vi "TIFF_6_Full_Write_Metadata.vi"(0 "Source File Image Path":path=path "C:/Users/Sebastien/Documents/GitHub/LABVIEW-Useful-codes/TIFF/Test_Image_1.tif", 5 "Destination Image Path":path=path "C:/Users/Sebastien/Documents/GitHub/LABVIEW-Useful-codes/TIFF/Test_Image_1_New.tif", 7 "User":T1(ring), 9 "XY resolution (nm)":string="125", 11 "error in (no error)":errorcluster) -> (15 "Error Out":errorcluster)   [LabVIEW 2025]
doc: "This software was created to prototype writing metadata to a TIFF file with a single image.\n\n<B>Usage:</B> This software is free to use, copy or plagiariaze. It is provided \"as-is\", and no technical support will be provided. The copyright is retained by NASA Marshall Space Flight Center.\n\n<B>Testing:</B> This software was tested by A) verifying that operations were completed successfully using LabVIEW 2009 on Windows XP, .NET version 4.0 and B) Windows Vista Microsoft Office Picture Manager was able to read and display the output file and C) Windows Vista Windows Photo Gallery was able to read and display the output file and the Description and D) Adobe Photoshop for Macintosh was able to correctly load and display the image and all the metadata.\n\n<B>Note:</B> This software requires .NET version 4.0\n\n<B>Warning:</B> This software will overwrite the destination file if it exists.\n\nThis software originally developed by:\nDerek Mayer\nBAE Systems - Technology Solutions & Services\n308 Voyager Way\nHuntsville, AL 35806\n(256) 890-8000\nwww.mevatec.com\nwww.baesystems.com/TSS\nSeptember 2010"
uses:
  TypeDef_FGV.ctl
  <vilib>/addons/_JKI.lib/Serialization/JSON/JKI JSON Serialization.lvlib
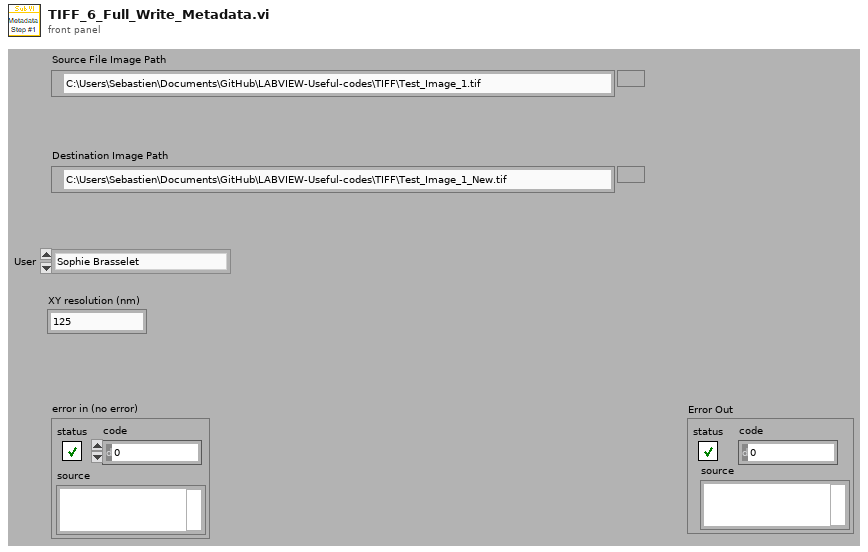
[diagram p1: front panel]
types:
  T1 = enum16{"Sophie Brasselet", "Jean-Jacques Honorine", "Sébastien Mailfert", "Manos Mavrakis"}
  T2 = typedef "TypeDef_FGV.ctl" = enum16{"Initialize", "Write", "Read", "Read_File", "Write_to_File"}
  T3 = typedef "TypeDef_Array_ChannelCluster.ctl" = cluster{"Laser":enum16{"640 nm", "561 nm"}, "Power":u8, "Exposure time":dbl, "Channel ON-OFF":bool, "Polar ON-OFF":bool, "FW 1":u16, "FW 2":u16}[]
  T4 = cluster{"Date/Time":string, "System model":string, "Software version":string, "Copyright":string, "User":string, "Description":string, "X resolution":string, "Y resolution":string, "Resolution unit":string}
  T5 = cluster{"Error":errorcluster, "Source Filestream":refnum<k24>, "TIFF Decoder":refnum<k24>, "TIFF Frames":refnum<k24>, "get_Item":refnum<k24>, "Bitmap Metadata":refnum<k24>, "New Encoder":refnum<k24>}
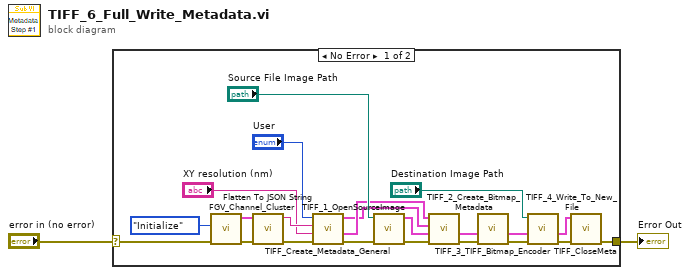
[diagram p0: block diagram]
diagram:
  n1 = case shown="No Error" "error in (no error)" {
    selector: "error in (no error)" -> [w12 w25]
    tunnel: [w14 w25] -> w1
    frame No Error {
      n2 = call "FGV_Channel_Cluster.vi"("error in"=w12, "Action"=TypeDef_FGV."Initialize") -> ("error out"=w11:errorcluster, "Channel_Cluster_Array OUT"=w10:T3)  [unwired: 8 in]
      n3 = call <vilib>:"Flatten To JSON String.vi"("error in"=w11, "Variant"=w10) -> ("error out"=w6:errorcluster, "JSON String"=w9:string)  [unwired: 8 in]
      n4 = call "TIFF_Create_Metadata_General.vi"("error in (no error)"=w6, "XY resolution (nm)"="XY resolution (nm)", "Description"=w9, "User"="User") -> ("error out"=w5:errorcluster, "Metadata OUT"=w4:T4, "Taggs"=w3:T4)  [unwired: 5 in]
      n5 = call "TIFF_1_OpenSourceImage.vi"("error in (no error)"=w5, "Source File Image Path"="Source File Image Path") -> ("Error Out"=w23:errorcluster, "output cluster"=w22:T5)  [unwired: 8 in]
      n6 = call "TIFF_2_Create_Bitmap_Metadata.vi"("error in (no error)"=w23, "Input cluster"=w22, "Taggs"=w3, "Metadata IN"=w4) -> ("Error Out"=w19:errorcluster, "Output cluster"=w20:T5)  [unwired: 6 in]
      n7 = call "TIFF_3_TIFF_Bitmap_Encoder.vi"("error in (no error)"=w19, "Cluster"=w20) -> ("Error Out"=w18:errorcluster, "output cluster"=w17:T5)  [unwired: 8 in]
      n8 = call "TIFF_4_Write_To_New_File.vi"("error in (no error)"=w18, "Input cluster"=w17, "Destination Image Path"="Destination Image Path") -> ("Error Out"=w15:errorcluster, "output cluster"=w16:T5)  [unwired: 7 in]
      n9 = call "TIFF_CloseMeta.vi"("error in (no error)"=w15, "Input cluster"=w16) -> ("error out"=w14:errorcluster)  [unwired: 9 in]
    }
    frame Error {
    }
  }
  "Error Out" <- w1
